vi "Is Concrete Class.vi"(0 "Scalar Path Group in":refnum<class "Scalar Path Group.lvclass">, 11 "error in (no error)":errorcluster) -> (4 "Scalar Path Group out":refnum<class "Scalar Path Group.lvclass">, 6 "Is Concrete Class?":bool, 15 "error out":errorcluster)   [LabVIEW 2023, in "RFFixtureCharact.Public.lvlib" / "Scalar Path Group.lvclass"]
uses:
  Scalar Path Group.lvclass
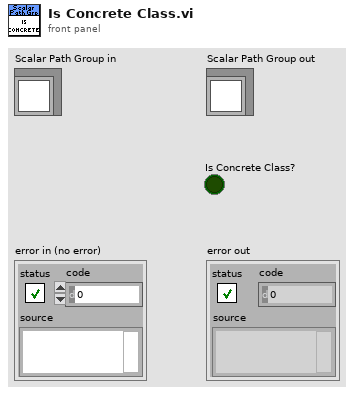
[diagram p1: front panel]
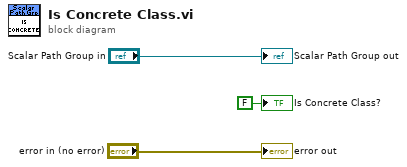
[diagram p0: block diagram]
diagram:
  "error out" <- "error in (no error)"
  "Scalar Path Group out" <- "Scalar Path Group in"
  "Is Concrete Class?" <- FALSE ("Is Concrete Class?")
